vi "Init Instruments.vi"(8 "error in (no error)":errorcluster, 10 "Physical Instr CFGs":string[](array[string]), 11 "IMSS Target Actor in":refnum<class "IMSS Target Actor.lvclass">) -> (0 "error out":errorcluster, 3 "IMSS Target Actor out":refnum<class "IMSS Target Actor.lvclass">)   [LabVIEW 2023, in "IMSS Target Actor.lvlib" / "IMSS Target Actor.lvclass"]
uses:
  IMSS Target Actor.lvclass
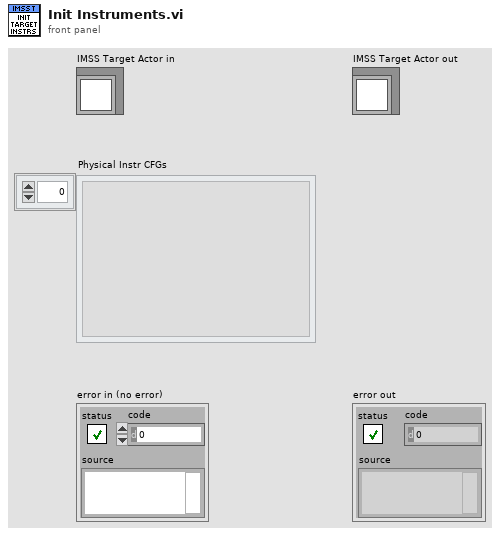
[diagram p1: front panel]
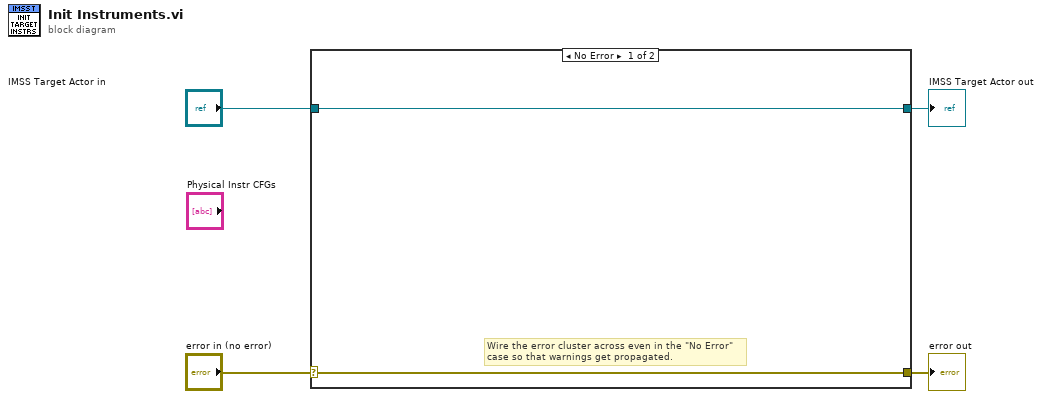
[diagram p0: block diagram]
diagram:
  n1 = case shown="No Error" "error in (no error)" {
    selector: "error in (no error)" -> [w5 w8]
    tunnel: [w5 w8] -> w3
    tunnel: [w6 w7] -> w1
    tunnel: "IMSS Target Actor in" -> [w6 w7]
    frame No Error {
      # "Wire the error cluster across even in the \"No Error\"\ncase so that warnings get propagated."
    }
    frame Error {
    }
  }
  "error out" <- w3
  "IMSS Target Actor out" <- w1
